vi "GetPosition.vi"(8 "error in (no error)":errorcluster, 11 "3D Object in":refnum<class "3D Object.lvclass">) -> (0 "error out":errorcluster, 2 "Position":cluster{"X":sgl, "Y":sgl, "Z":sgl}, 3 "3D Object out":refnum<class "3D Object.lvclass">)   [LabVIEW 2015, in "3D Object.lvclass"]
uses:
  3D Object.lvclass
  3D Object.lvclass/3D Object.ctl
  <vilib>/picture/3D Picture Control/NI_3D Picture Control.lvlib
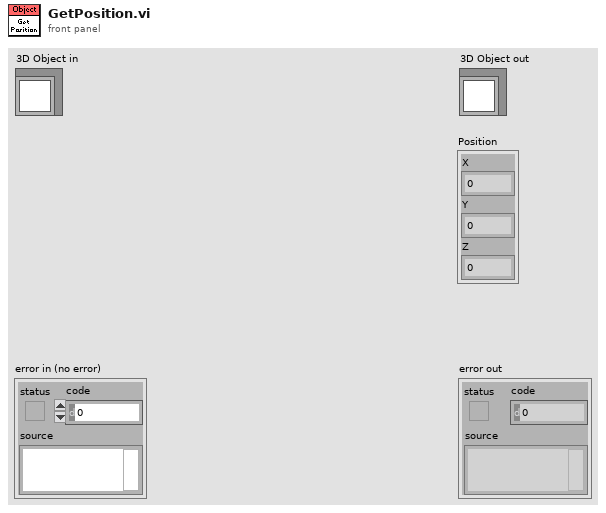
[diagram p1: front panel]
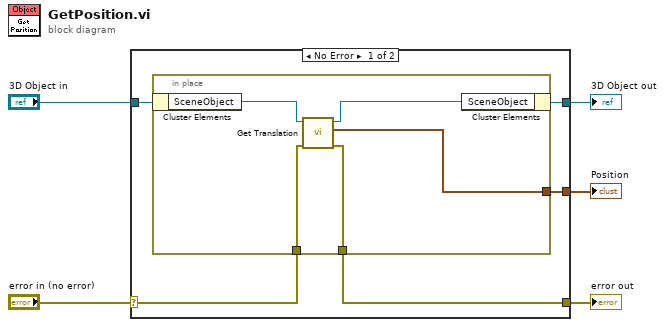
[diagram p0: block diagram]
diagram:
  n1 = case shown="No Error" "error in (no error)" {
    selector: "error in (no error)" -> [w7 w16]
    tunnel: [w6 w16] -> w4
    tunnel: [w9 w17] -> w2
    tunnel: "3D Object in" -> [w10 w17]
    tunnel: [w8 _] -> w1
    frame No Error {
      n2 = in-place {
        in-place-border: [w13] -> w8
        in-place-border: w7 -> [w12]
        in-place-border: [w11] -> w6
        n3 = in-place-cluster #1(w10) -> ("SceneObject"=w15:refnum<vi>)
        n4 = call <vilib>:"Get Translation.vi"("error in (no error)"=w12, "Scene Object"=w15) -> ("error out"=w11:errorcluster, "Transformation:Get Translation"=w13:cluster{"X":sgl, "Y":sgl, "Z":sgl}, "Scene Object"=w14:refnum<vi>)  [unwired: 7 in]
        n5 = in-place-cluster #1("SceneObject"=w14) -> (w9:refnum<class "3D Object.lvclass">)
      }
    }
    frame Error {
    }
  }
  "error out" <- w4
  "3D Object out" <- w2
  "Position" <- w1
